vi "Get Tag Symbol.vi"(8 "error in (no error)":errorcluster, 11 "Tag_LVOOP in":refnum<class "Tree Tag Class.lvclass">) -> (0 "error out":errorcluster, 2 "Symbol Index":i32, 3 "Tag_LVOOP out":refnum<class "Tree Tag Class.lvclass">)   [LabVIEW 2012, in "Tree Tools.lvlib" / "Tree Tag Class.lvclass"]
uses:
  Tree Tag Class.lvclass
  Tree Tag Class.lvclass/Tree Tag Class.ctl
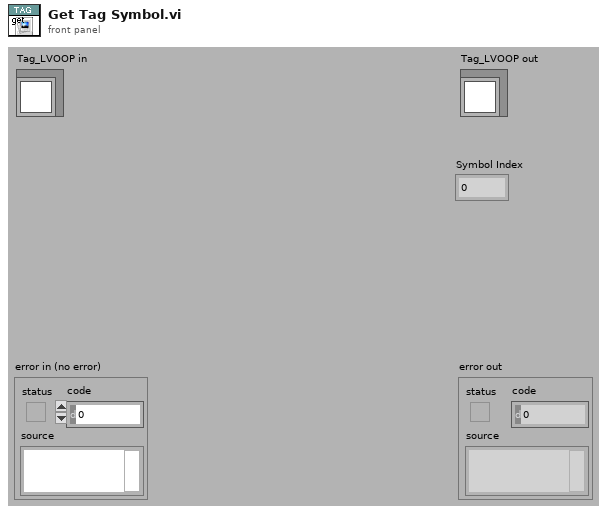
[diagram p1: front panel]
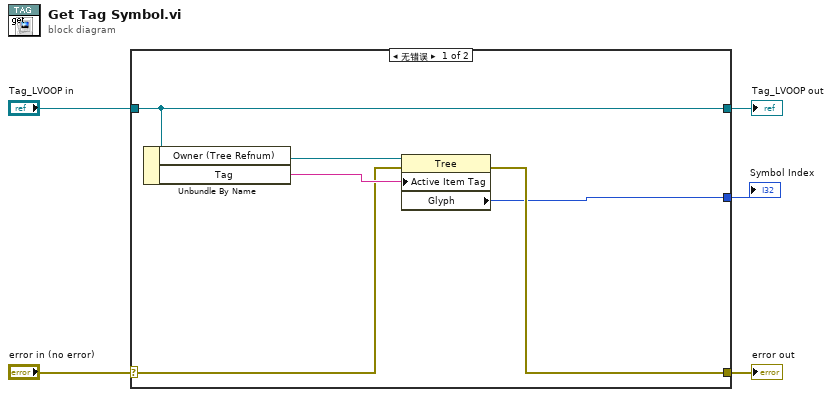
[diagram p0: block diagram]
diagram:
  n1 = case shown="无错误" "error in (no error)" {
    selector: "error in (no error)" -> [w8 w13]
    tunnel: [w7 w13] -> w4
    tunnel: [w11 w12] -> w2
    tunnel: "Tag_LVOOP in" -> [w11 w12]
    tunnel: [w6 _] -> w1
    frame No Error {
      n2 = Unbundle By Name(w11) -> ("Owner (Tree Refnum)"=w10:refnum<vi>, "Tag"=w9:string)
      n3 = property class="Tree"(reference=w10, error in=w8, "Active Item Tag"=w9) -> (error out=w7:errorcluster, "Glyph"=w6:i32)  [unwired: 1 out]
    }
    frame Error {
    }
  }
  "error out" <- w4
  "Tag_LVOOP out" <- w2
  "Symbol Index" <- w1
